vi "Temporary Filename__ogtk.vi"(4 "error in (no error)":errorcluster, 6 "pattern (lvtemp%d.tmp)":string, 7 "sub directory":path=path "") -> (0 "error out":errorcluster, 3 "file in tmp dir":path)   [LabVIEW 2016]
doc: "Generates an unused temporary file path."
panel:
  # "Temporary Filename.vi\n\nGenerates an unused temporary file path.\n\nPlease visit http://www.OpenG.org to learn about the\nOpen Source LabVIEW software movement.\n\nNOTICE -- YOU MUST LEAVE THIS NOTICE IN PLACE.  PER THE TERMS OF THE LICENSE BELOW, YOU MAY SUBLICENSE THIS SOFTWARE \nIN ANY WAY THAT DOES NOT CONFLICT WITH THIS LICENSE.\n\n### BSD License (http://www.opensource.org/licenses/bsd-license.php) Begin ###\n\nCopyright (c) 2004, Rolf Kalbermatter <rolf.kalbermatter@citeng.com>\nCopyright (c) 2006, Jim Kring <jim@jimkring.com>\n\nAll rights reserved.\n\nRedistribution and use in source and binary forms, with or without modification, are permitted provided that the following conditions are met:\n\n    * Redistributions of source code must retain the above copyright notice, this list of conditions and the following disclaimer.\n    * Redistributions in binary form must reproduce the above copyright notice, this list of conditions and the following disclaimer in the \n       documentation and/or other materials provided with the distribution.\n    * Neither the name of SciWare, James Kring, Inc., nor the names of its contributors may be used to endorse or promote products derived \n       from this software without specific prior written permission.\n\nTHIS SOFTWARE IS PROVIDED BY THE COPYRIGHT HOLDERS AND CONTRIBUTORS \"AS IS\" AND ANY EXPRESS OR IMPLIED WARRANTIES, \nINCLUDING, BUT NOT LIMITED TO, THE IMPLIED WARRANTIES OF MERCHANTABILITY AND FITNESS FOR A PARTICULAR PURPOSE ARE \nDISCLAIMED. IN NO EVENT SHALL THE COPYRIGHT OWNER OR CONTRIBUTORS BE LIABLE FOR ANY DIRECT, INDIRECT, INCIDENTAL,\n SPECIAL, EXEMPLARY, OR CONSEQUENTIAL DAMAGES (INCLUDING, BUT NOT LIMITED TO, PROCUREMENT OF SUBSTITUTE GOODS OR \nSERVICES; LOSS OF USE, DATA, OR PROFITS; OR BUSINESS INTERRUPTION) HOWEVER CAUSED AND ON ANY THEORY OF LIABILITY, \nWHETHER IN CONTRACT, STRICT LIABILITY, OR TORT (INCLUDING NEGLIGENCE OR OTHERWISE) ARISING IN ANY WAY OUT OF THE USE \nOF THIS SOFTWARE, EVEN IF ADVISED OF THE POSSIBILITY OF SUCH DAMAGE.\n\n### BSD License End ###"
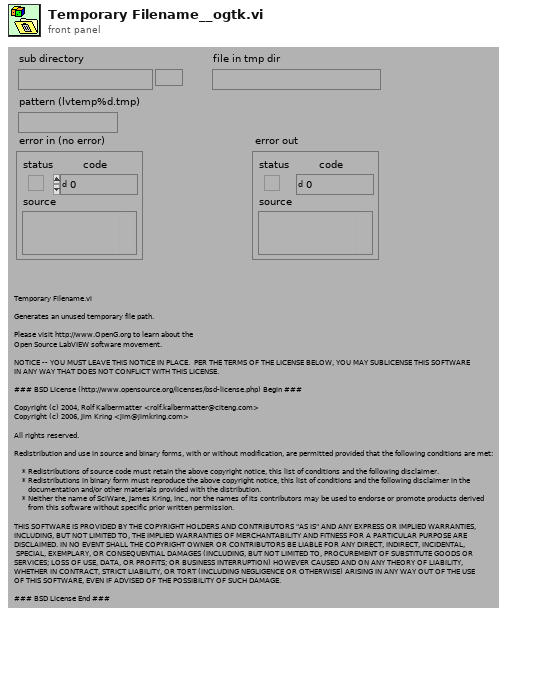
[diagram p1: front panel]
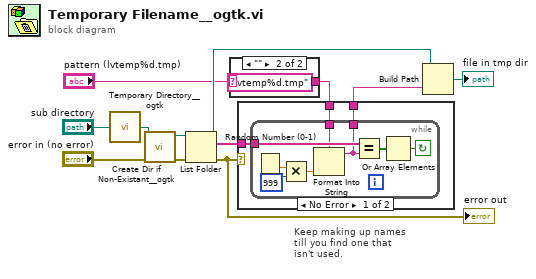
[diagram p0: block diagram]
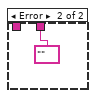
[diagram p2: hidden frame]
diagram:
  # "Keep making up names\ntill you find one that\nisn't used."
  n1 = call <userlib>:"Temporary Directory__ogtk.vi"("Relative path (.)"="sub directory") -> ("Temporary Directory (+ Relative)"=w7:path)
  n2 = call <userlib>:"Create Dir if Non-Existant__ogtk.vi"("error in (no error)"="error in (no error)", "Directory Path"=w7) -> ("error out"=w5:errorcluster, "dup Directory Path"=w6:path)  [unwired: 7 in, 1 out]
  n3 = List Folder(path=w6, error in=w5) -> (path out=w8:path, filenames=w12:string[], error out=w1:errorcluster)  [unwired: 2 in, 1 out]
  "error out" <- w1
  n4 = case shown="\"\"" "pattern (lvtemp%d.tmp)" {
    selector: "pattern (lvtemp%d.tmp)" -> [w13 _]
    tunnel: [w13 "lvtemp%d.tmp" ("pattern (lvtemp%d.tmp)")] -> w2
    frame Default {
    }
    frame "" {
    }
  }
  n5 = case shown="No Error" w1 {
    tunnel: w12 -> [w17 _]
    tunnel: [w16 ""] -> w11
    tunnel: w2 -> [w15 _]
    frame No Error {
      n6 = while {
        tunnel: [w18] -> w16
        tunnel: w17 -> [w23]
        tunnel: w15 -> [w20]
        stop <- w21 continue-if-true
        n7 = Random Number (0-1)() -> (number: 0 to 1=w24:dbl)
        n8 = Multiply(x=w24, y=999) -> (x*y=w19:dbl)
        n9 = Format Into String(format string=w20, w19) -> (resulting string=w18:string)  [unwired: 2 in, 1 out]
        n10 = Equal?(x=w23, y=w18) -> (x = y?=w22:bool[])
        n11 = Or Array Elements(Boolean array=w22) -> (logical OR=w21:bool)
      }
    }
    frame Error {
    }
  }
  n12 = Build Path(base path=w8, name or relative path=w11) -> (appended path=→"file in tmp dir":path)
